vi "DAQ-Stop All.vi"(11 "error in (no error)":errorcluster) -> (15 "error out":errorcluster)   [LabVIEW 2020]
uses:
  AIDI/Typedefs/AIDI-Action.ctl
  AODO/Typedefs/AODO-Action.ctl
  Counter/Typedefs/CTR-Action.ctl
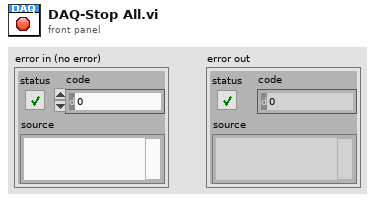
[diagram p1: front panel]
types:
  T1 = typedef "CTR-Action.ctl" = enum16{"Clear", "Configure", "Initialize", "Init & Start", "Start", "Clean up"}
  T2 = typedef "AODO-Action.ctl" = enum16{"Configure", "Initialize", "Start", "Write", "Clean up", "Init & Start", "Config & Test", "Position", "Set AO Gains", "Zero", "Prime", "Status"}
  T3 = typedef "AIDI-Action.ctl" = enum16{"Configure", "Initialize", "Start", "Read", "Clean up", "Init & Start", "Config & Test", "Position", "Skip"}
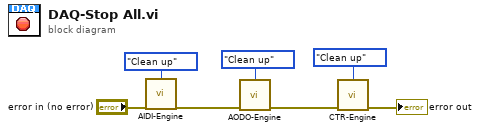
[diagram p0: block diagram]
diagram:
  n1 = call "AIDI-Engine.vi"("Action"=AIDI-Action."Clean up", "error in (no error)"="error in (no error)") -> ("error out"=w6:errorcluster)  [unwired: 8 in, 5 out]
  n2 = call "AODO-Engine.vi"("Action"=AODO-Action."Clean up", "error in (no error)"=w6) -> ("error out"=w3:errorcluster)  [unwired: 9 in, 4 out]
  n3 = call "CTR-Engine.vi"("action"=CTR-Action."Clean up", "error in (no error)"=w3) -> ("error out"=→"error out":errorcluster)  [unwired: 13 in]
